vi "TimerDRV Tester.vi"() -> ()   [LabVIEW 2019, in "TimingDRV Engine.lvlib"]
uses:
  TimingDRV Engine.lvlib
  TypeDefs/Target Type.ctl
  <vilib>/Platform/TimedLoop/XDataNode/timing_clust.ctl
  <vilib>/Platform/TimedLoop/XDataNode/nitl_modes.ctl
  <vilib>/Platform/TimedLoop/XDataNode/wakeup.ctl
  <vilib>/Platform/TimedLoop/scheduler/LVUserAPI/_suppVIs/Create_SoftwareTrigger_TSource.vi
  Methods/Configure TimerDRV Instances/Configure Controlled TimerDRV.vi
  <vilib>/platform/TimedLoop/XDataNode/XDataNode.xnode
  <vilib>/Platform/TimedLoop/XDataNode/XDNodeRunTimeDep.lvlib
  TimerDRV.lvclass
panel:
  in  "Trigger Loop Stop":bool
  in  "Trigger":bool
  out "Execution Speed":dbl[](graph)
  out "error out":errorcluster
  out "Execution Speed (Hz)":dbl
  in  "stop":bool
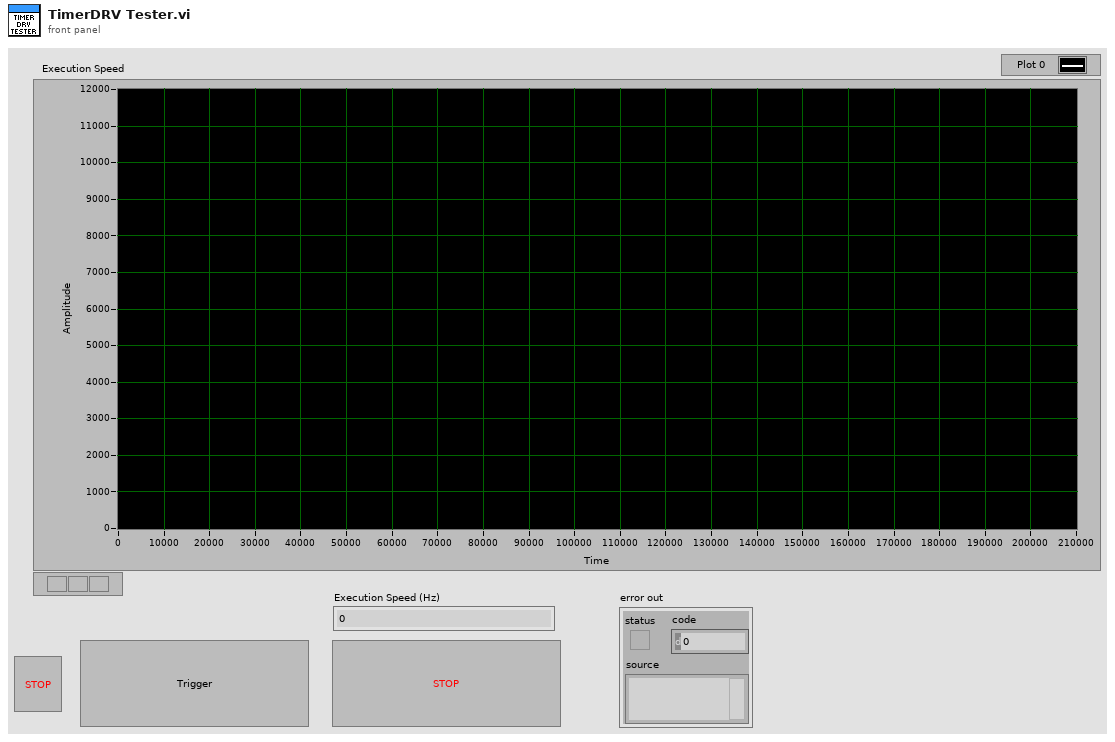
[diagram p1: front panel]
types:
  T1 = typedef "TimingDRV Engine.lvlib/TimerDRV.lvclass/Target Type.ctl" = enum16{"PharLap", "VxWorks", "Windows", "Linux_32_ARM", "Linux_x64"}
  T2 = typedef "XDNodeRunTimeDep.lvlib/timing_clust.ctl" = cluster{"Expected End [f-1]":u64, "Actual End [f-1]":u64, "Finished Late? [f-1]":bool, "Expected End [i-1]":u64, "Actual End [i-1]":u64, "Finished Late? [i-1]":bool, "Expected Start [i]":u64, "Actual Start [i]":u64, "Expected Start [f]":u64, "Actual Start [f]":u64, "Source Name":string, "Structure Name":string, "Period":i64, "Deadline":i64, "Offset":i64, "Start":i64, "Priority":i32, "Timeout":i32, "Mode":T3, "Wakeup Reason":T4, "Error":errorcluster, "Source Type":string, "Secondary Source Type":string, "Global End Time":u64, "Global Start Time":u64, "Frame Duration":u64, "Iteration Duration":u64, "Assigned CPU":i32, "I/O Scan Engine Mode":u32}
  T3 = typedef "XDNodeRunTimeDep.lvlib/nitl_modes.ctl" = enum32{"No Change", "Process missed periods, maintain original phase", "Discard missed periods, maintain original phase", "Process missed periods, ignore original phase", "Discard missed periods, ignore original phase"}
  T4 = typedef "XDNodeRunTimeDep.lvlib/wakeup.ctl" = enum32{"Normal", "Aborted", "Asynchronous wakeup", "Timing source error", "Timed loop error", "Timeout"}
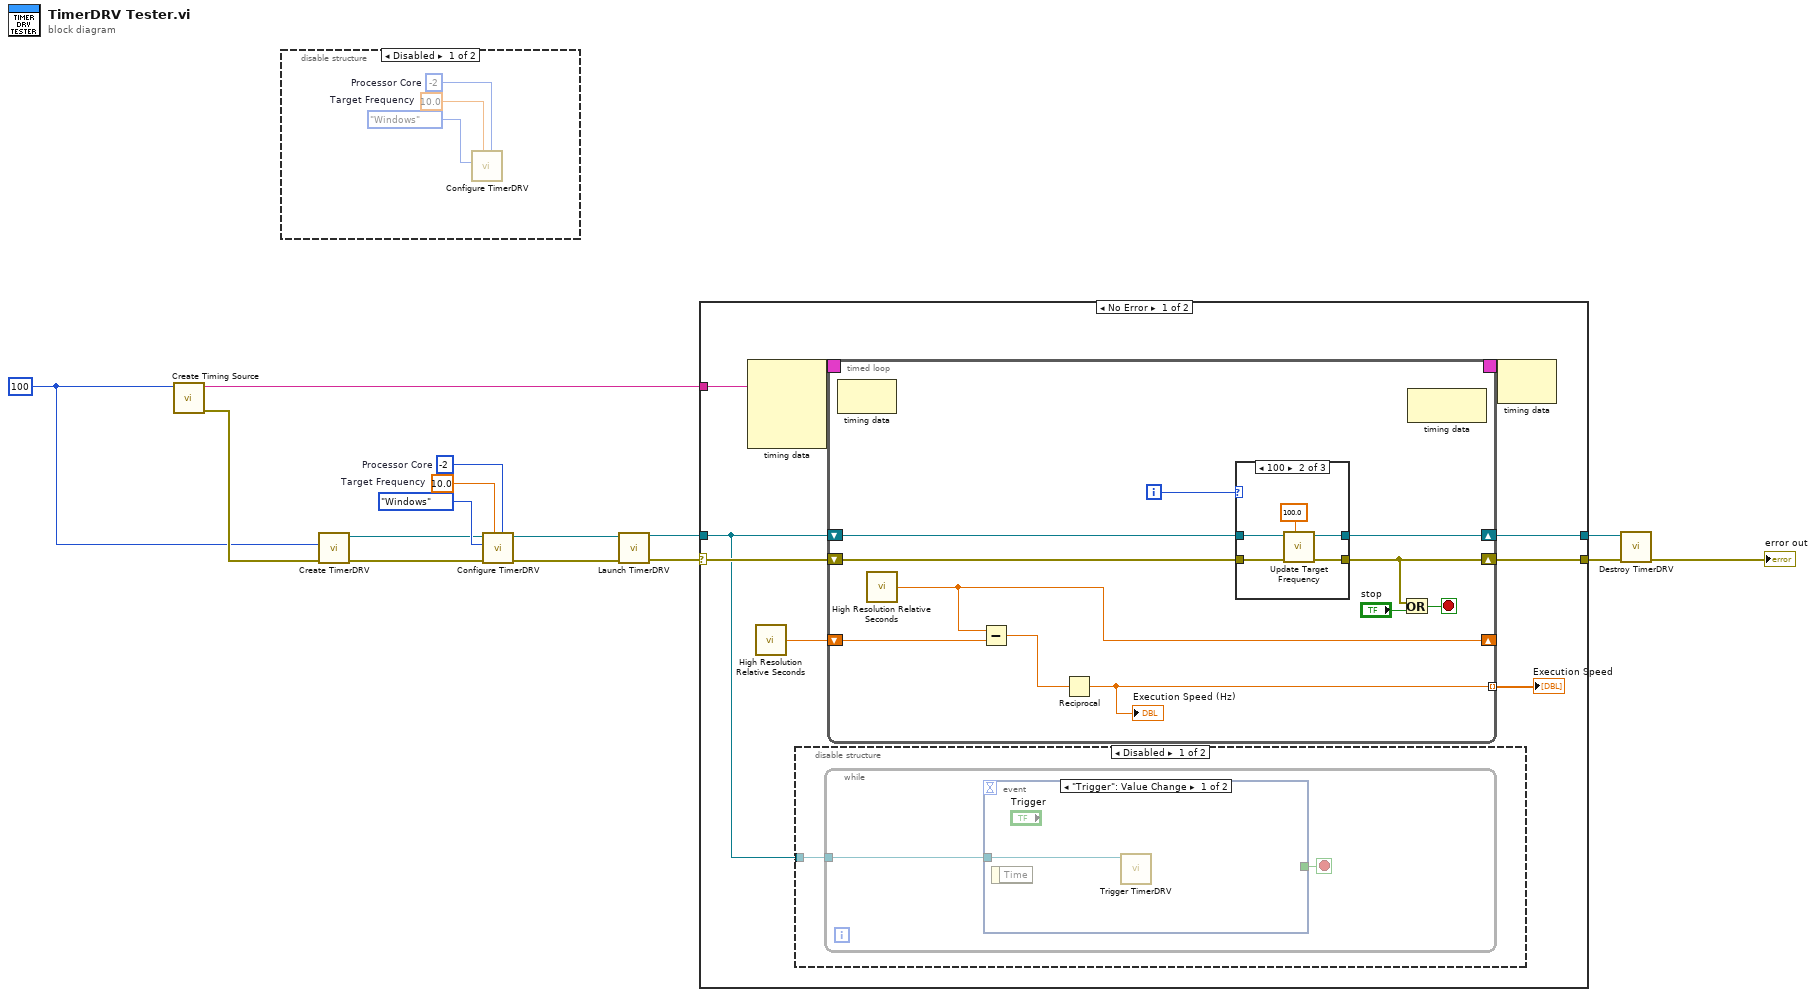
[diagram p0: block diagram]
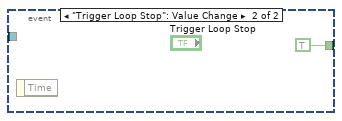
[diagram p3: hidden frame]
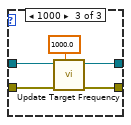
[diagram p6: hidden frame]
diagram:
  w7 = -2  # Processor Core
  w6 = 10.0  # Target Frequency
  w13 = u8 100 ("Trigger ID")
  n1 = call-poly <vilib>:"Create Timing Source.vi"("trigger ID"=w13) -> ("error out"=w14:errorcluster, "timing source name"=w15:string)  [unwired: 9 in]
  n2 = disable-structure shown="Disabled" {
    frame Disabled {
      w16 = -2  # Processor Core
      w17 = 10.0  # Target Frequency
      n3 = call-poly "Configure TimerDRV.vi"("Processor Core"=w16, "Target Frequency"=w17, "Target Type"=Target_Type."Windows") -> ()  [unwired: 7 in, 2 out]
    }
    frame Enabled {
    }
  }
  n4 = call "Create TimerDRV.vi"("error in (no error)"=w14, "Trigger ID"=w13) -> ("error out"=w4:errorcluster, "TimerDRV out"=w3:refnum<class "TimerDRV.lvclass">)  [unwired: 8 in]
  n5 = call-poly "Configure TimerDRV.vi"("Processor Core"=w7, "Target Frequency"=w6, "error in (no error)"=w4, "Target Type"=Target_Type."Windows", "TimerDRV in"=w3) -> ("error out"=w1:errorcluster, "TimerDRV out"=w2:refnum<class "TimerDRV.lvclass">)  [unwired: 5 in]
  n6 = call "Launch TimerDRV.vi"("error in (no error)"=w1, "TimerDRV in"=w2) -> ("error out"=w11:errorcluster, "TimerDRV out"=w12:refnum<class "TimerDRV.lvclass">)  [unwired: 8 in]
  n7 = case shown="No Error" w11 {
    selector: w11 -> [w21 w62]
    tunnel: w12 -> [w19 w63]
    tunnel: [w25 w62] -> w10
    tunnel: [w24 w63] -> w8
    tunnel: w15 -> [w23 _]
    frame No Error {
      n8 = node-c288(w23) -> (w27:T2)  [unwired: 3 in]
      n9 = call <vilib>:"High Resolution Relative Seconds.vi"() -> ("relative seconds"=w22:dbl)
      n10 = disable-structure shown="Disabled" {
        disable-tunnel: w19 -> [w28 _]
        frame Disabled {
          n11 = while {
            tunnel: w28 -> [w30]
            stop <- w29 stop-if-true
            n12 = event shown="[0] \"Trigger\": Value Change" {
              selector: _ -> [_ _]
              dyn-events: _ -> [_ _]
              timeout: _ -> [_ _]
              tunnel: w30 -> [w31 _]
              tunnel: [_ TRUE] -> w29
              event "Trigger": Value Change {
                n13 = event-data() -> ()  [unwired: 1 in, 1 out]
                n14 = call "Trigger TimerDRV.vi"("TimerDRV in"=w31) -> ()  [unwired: 9 in, 2 out]
              }
              event "Trigger Loop Stop": Value Change {
                n15 = event-data() -> ()  [unwired: 1 in, 1 out]
              }
            }
          }
        }
        frame Enabled {
        }
      }
      n16 = timed-loop {
        shift-right: [w37] -> w24
        shift-left: w19 -> [w39]
        shift-right: [w34] -> w25
        shift-left: w21 -> [w38]
        timing: w27 -> [_]
        timing-out: [_] -> w26
        shift-right: [w42] -> _
        shift-left: w22 -> [w43]
        tunnel: [w33] -> w20 mode=indexing
        i -> [w40]
        stop <- w36 stop-if-true
        n17 = node-c288() -> ()  [unwired: 1 in, 1 out]
        n18 = call <vilib>:"High Resolution Relative Seconds.vi"() -> ("relative seconds"=w42:dbl)
        n19 = Subtract(x=w42, y=w43) -> (x-y=w41:dbl)
        n20 = Reciprocal(x=w41) -> (1/x=w33:dbl)
        "Execution Speed (Hz)" <- w33
        n21 = case shown="100" w40 {
          tunnel: w39 -> [w45 w49 w54]
          tunnel: w38 -> [w44 w50 w55]
          tunnel: [w45 w47 w52] -> w37
          tunnel: [w44 w48 w53] -> w34
          frame 0, Default {
          }
          frame 100 {
            n22 = call "Update Target Frequency.vi"("New Target Frequency"=100.0 ("Target Frequency"), "error in (no error)"=w50, "TimerDRV in"=w49) -> ("error out"=w48:errorcluster, "TimerDRV out"=w47:refnum<class "TimerDRV.lvclass">)  [unwired: 7 in]
          }
          frame 1000 {
            n23 = call "Update Target Frequency.vi"("New Target Frequency"=1000.0 ("Target Frequency"), "error in (no error)"=w55, "TimerDRV in"=w54) -> ("error out"=w53:errorcluster, "TimerDRV out"=w52:refnum<class "TimerDRV.lvclass">)  [unwired: 7 in]
          }
        }
        n24 = Or(x=w34, y="stop") -> (x .or. y?=w36:bool)
        n25 = node-c288() -> ()  [unwired: 1 in, 1 out]
      }
      "Execution Speed" <- w20
      n26 = node-c288(w26) -> ()  [unwired: 1 out]
    }
    frame Error {
    }
  }
  n27 = call "Destroy TimerDRV.vi"("error in (no error)"=w10, "TimerDRV in"=w8) -> ("error out"=→"error out":errorcluster)  [unwired: 9 in]
